vi "Test Verify.vi"(11 "Test Case In":refnum<class "Core Library Error Propagation.lvclass">) -> (0 "error out":errorcluster, 3 "Test Case Out":refnum<class "Core Library Error Propagation.lvclass">)   [LabVIEW 2020, in "Core Library Error Propagation.lvclass"]
uses:
  Core Library Error Propagation.lvclass
  Source/Approval Tests/Options/Options.lvclass
  Source/Approval Tests/Scrubber/Scrubber.lvclass
  Source/Approval Tests/Namer/Namer.lvclass
  Source/Approval Tests/Naming Data/Naming Data.lvclass
  Source/Approval Tests/Reporter/Reporter.lvclass
  Source/Approval Tests/Text Comparator/Text Comparator.lvclass
  <vilib>/Comparison/Equal/Equal Functor/Equal Functor.lvclass
  <vilib>/Astemes/LUnit/Palette/Advanced Assertions/LUnit Advanced Assertions.lvlib
  22289306-43b7-4406-bbac-392b8c610bd0.vi
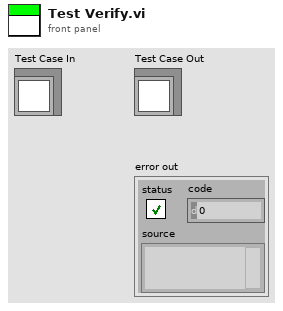
[diagram p1: front panel]
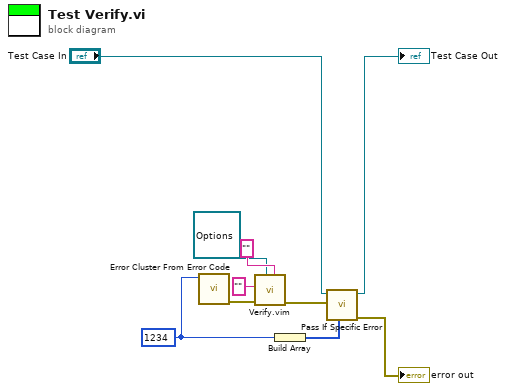
[diagram p0: block diagram]
diagram:
  w6 = 1234 ("error code (0)")
  n1 = call <vilib>:"Error Cluster From Error Code.vi"("error code (0)"=w6) -> ("error out"=w5:errorcluster)  [unwired: 8 in]
  n2 = call "Verify.vim"("Label"="", "Options"=refnum<class "Options.lvclass"> refnum, "error in"=w5, "Anything"="") -> ("error out"=w4:errorcluster)  [unwired: 5 in, 2 out]
  n3 = Build Array(w6) -> (w7:i32[])
  n4 = call <vilib>:"Pass If Specific Error.vi"("Error Codes"=w7, "Assert error"=w4, "LUnit Test Case In"="Test Case In") -> ("error out"=→"error out":errorcluster, "LUnit Test Case Out"=→"Test Case Out":refnum<class "Core Library Error Propagation.lvclass">)  [unwired: 7 in]
